vi "MinimalHost_FPGA_TEST.vi"() -> ()   [LabVIEW 2018]
uses:
  <vilib>/rvi/interface/nirviOpenFPGA/nirviOpenFPGA.xnode
  <vilib>/rvi/interface/nirviReadWriteControl/nirviReadWriteControl.xnode
  <vilib>/rvi/interface/Simulation/niFpgaSimulationCallBeginRW.vi
  <vilib>/rvi/errors/niLvFpgaAdjustHostInterfaceError.vi
  ProjectFiles/FPGA Bitfiles/FPGALoopCountTest_3.lvbitx
  TestCode/FPGA_LoopCount_Test.vi
panel:
  out "error out 2":errorcluster
  out "Configuration Error 2":bool
  out "Configured? 2":bool
  out "SPI Idle":bool
  out "LoopCount":i32
  out "error out":errorcluster
  out "IO Module\\Initialization Done":bool
  out "FPGA Probe":i16
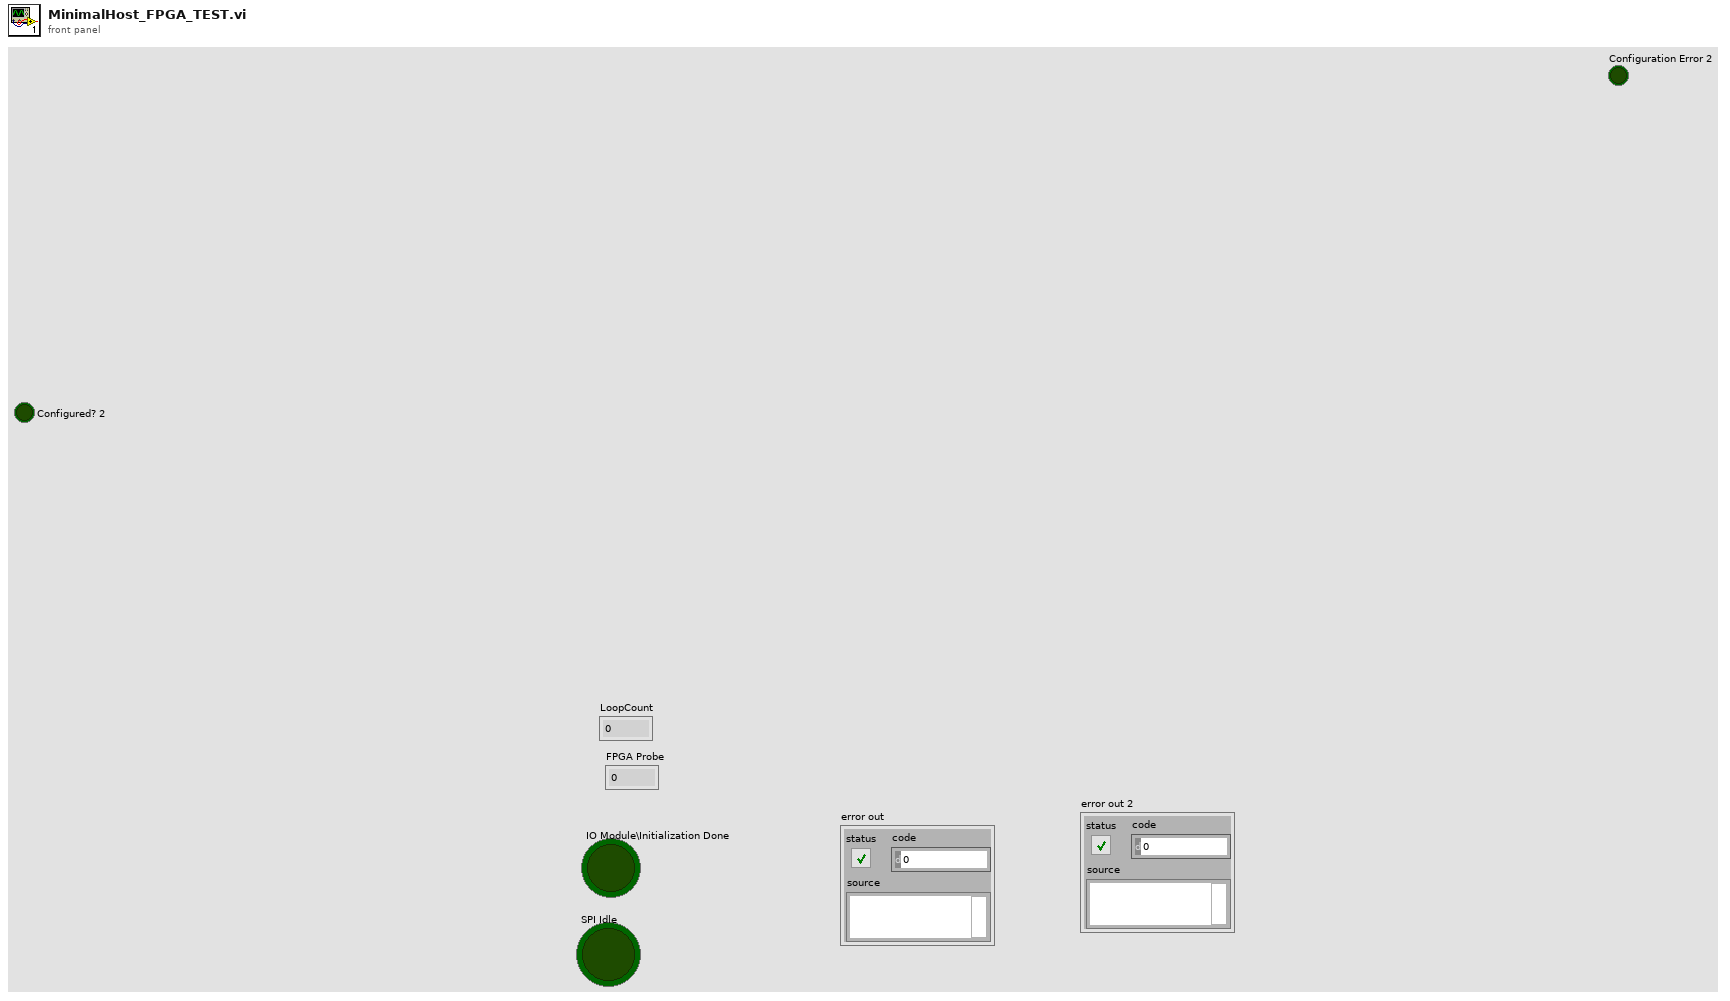
[diagram p1: front panel]
types:
  T1 = enum8{"Internal Clock PLL Off", "Internal Clock PLL On (CLK_IN)", "External Clock (CLK_IN)", "Internal Clock PLL On (IoModSyncClk)"}
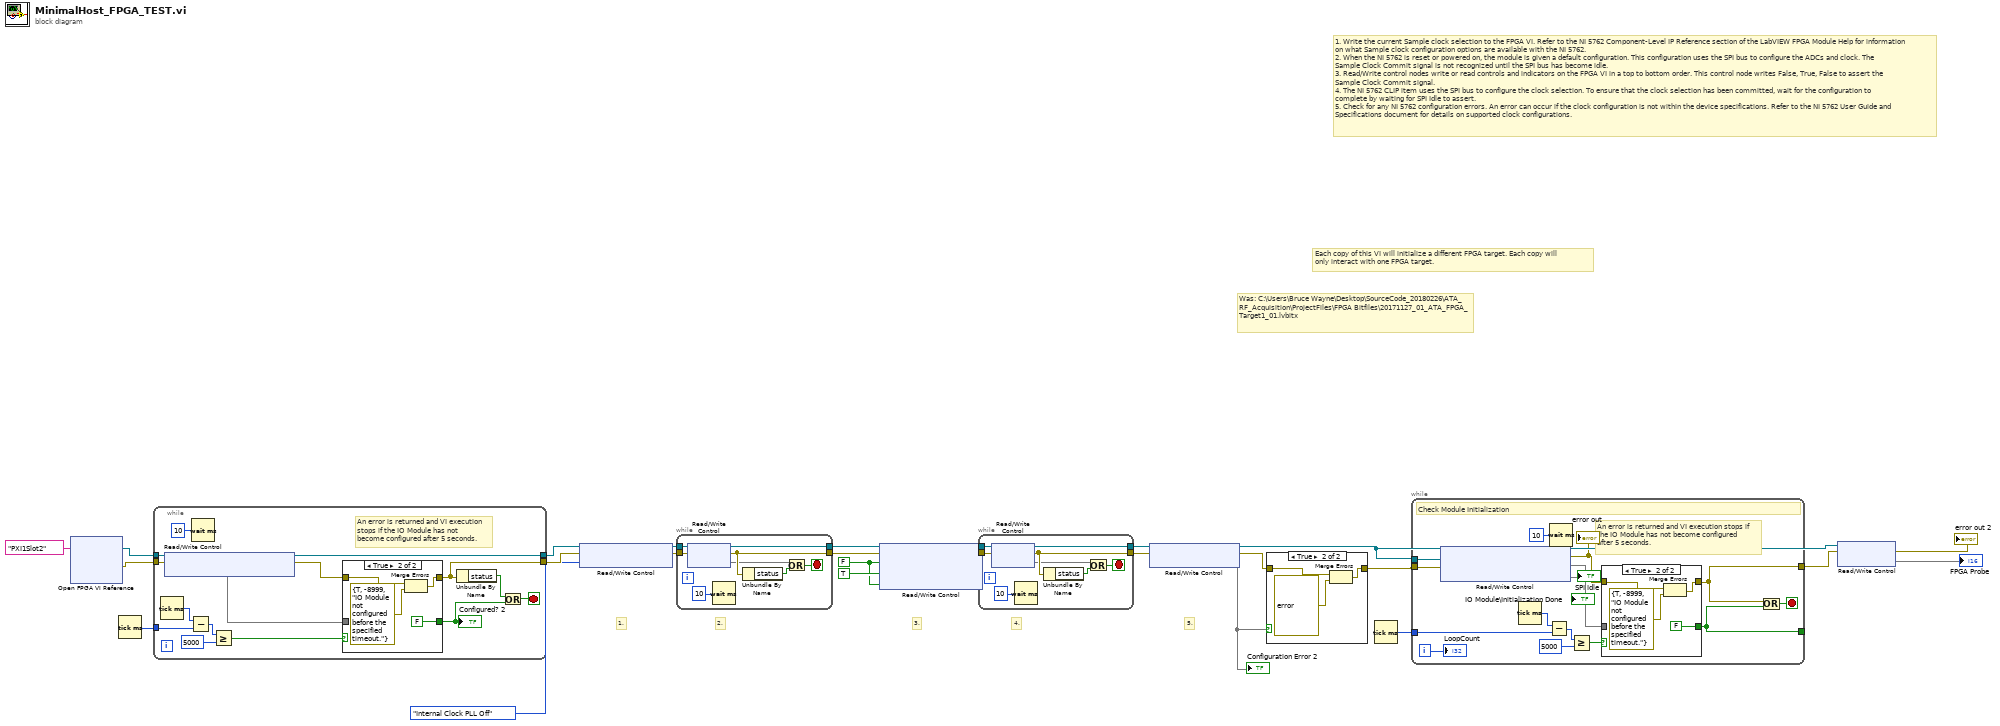
[diagram p0: block diagram]
diagram:
  w15 = FALSE ("Sample Clock Commit")
  # "1. Write the current Sample clock selection to the FPGA VI. Refer to the NI 5762 Component-Level IP Reference section of the LabVIEW FPGA Module Help for information on what Sample clock configuration options are available with the NI 5762.\n2. When the NI 5762 is reset or powered on, the module is given a default configuration. This configuration uses the SPI bus to configure the ADCs and clock. The Sample Clock Commit signal is not recognized until the SPI bus has become idle.\n3. Read/Write control nodes write or read controls and indicators on the FPGA VI in a top to bottom order. This control node writes False, True, False to assert the Sample Clock Commit signal.\n4. The NI 5762 CLIP item uses the SPI bus to configure the clock selection. To ensure that the clock selection has been committed, wait for the configuration to complete by waiting for SPI Idle to assert.\n5. Check for any NI 5762 configuration errors. An error can occur if the clock configuration is not within the device specifications. Refer to the NI 5762 User Guide and Specifications document for details on supported clock configurations."
  # "5."
  # "4."
  # "3."
  # "2."
  # "1."
  # "Was: C:\\Users\\Bruce Wayne\\Desktop\\SourceCode_20180226\\ATA_RF_Acquisition\\ProjectFiles\\FPGA Bitfiles\\20171127_01_ATA_FPGA_Target1_01.lvbitx"
  # "Each copy of this VI will initialize a different FPGA target. Each copy will\nonly interact with one FPGA target."
  n1 = xnode ("Open FPGA VI Reference")("resource name"=tag "PXI1Slot2") -> ("FPGA VI Reference Out"=w8:refnum<k20>, "error out"=w7:errorcluster)  [unwired: 1 in]
  n2 = Tick Count (ms)() -> (millisecond timer value=w21:u32)
  n3 = while {
    tunnel: w7 -> [w33]
    tunnel: [w37] -> w6
    tunnel: [w29] -> w5
    tunnel: w8 -> [w32]
    tunnel: w21 -> [w27]
    stop <- w35 stop-if-true
    # "An error is returned and VI execution stops if the IO Module has not become configured after 5 seconds."
    n4 = Tick Count (ms)() -> (millisecond timer value=w28:u32)
    n5 = xnode "Read/Write Control"("FPGA VI Reference In"=w32, "error in"=w33) -> ("FPGA VI Reference Out"=w29:refnum<k20>, "error out"=w30:errorcluster, "IO Module\\Initialization Done"=w31)
    n6 = Subtract(x=w28, y=w27) -> (x-y=w26:u32)
    n7 = Wait (ms)(milliseconds to wait=u32 10) -> ()  [unwired: 1 out]
    n8 = Greater Or Equal?(x=w26, y=u32 5000) -> (x >= y?=w38:bool)
    n9 = case shown="True" w38 {
      tunnel: [w42 FALSE ("Configured?")] -> w34
      tunnel: w31 -> [w42 _]
      tunnel: [w41 w45] -> w37
      tunnel: w30 -> [w41 w43]
      frame False {
      }
      frame True {
        n10 = Merge Errors(w43, errorcluster {"status"=TRUE, "code"=-8999, "source"="IO Module not configured before the specified timeout."} ("error in")) -> (w45:errorcluster)
      }
    }
    "Configured? 2" <- w34
    n11 = Unbundle By Name(w37) -> ("status"=w36:bool)
    n12 = Or(x=w36, y=w34) -> (x .or. y?=w35:bool)
  }
  n13 = xnode "Read/Write Control"("FPGA VI Reference In"=w5, "error in"=w6, "Sample Clock Select"=T1."Internal Clock PLL Off" ("Clock Source 2")) -> ("FPGA VI Reference Out"=w9:refnum<k20>, "error out"=w10:errorcluster)
  n14 = while {
    tunnel: w9 -> [w50]
    tunnel: w10 -> [w51]
    tunnel: [w48] -> w12
    tunnel: [w49] -> w11
    stop <- w52 stop-if-true
    n15 = xnode "Read/Write Control"("FPGA VI Reference In"=w50, "error in"=w51) -> ("FPGA VI Reference Out"=w49:refnum<k20>, "error out"=w48:errorcluster, "SPI Idle"=w47)
    n16 = Wait (ms)(milliseconds to wait=u32 10) -> ()  [unwired: 1 out]
    n17 = Unbundle By Name(w48) -> ("status"=w53:bool)
    n18 = Or(x=w47, y=w53) -> (x .or. y?=w52:bool)
  }
  n19 = xnode "Read/Write Control"("FPGA VI Reference In"=w11, "error in"=w12, "Sample Clock Commit"=w15, "Sample Clock Commit"=TRUE, "Sample Clock Commit"=w15) -> ("FPGA VI Reference Out"=w13:refnum<k20>, "error out"=w14:errorcluster)
  n20 = while {
    tunnel: w13 -> [w59]
    tunnel: w14 -> [w58]
    tunnel: [w56] -> w18
    tunnel: [w57] -> w17
    stop <- w60 stop-if-true
    n21 = xnode "Read/Write Control"("FPGA VI Reference In"=w59, "error in"=w58) -> ("FPGA VI Reference Out"=w57:refnum<k20>, "error out"=w56:errorcluster, "SPI Idle"=w55)
    n22 = Wait (ms)(milliseconds to wait=u32 10) -> ()  [unwired: 1 out]
    n23 = Unbundle By Name(w56) -> ("status"=w61:bool)
    n24 = Or(x=w55, y=w61) -> (x .or. y?=w60:bool)
  }
  n25 = xnode "Read/Write Control"("FPGA VI Reference In"=w17, "error in"=w18) -> ("FPGA VI Reference Out"=w4:refnum<k20>, "error out"=w19:errorcluster, "Configuration Error"=w20)
  "Configuration Error 2" <- w20
  n26 = case shown="True" w20 {
    tunnel: [w63 w66] -> w3
    tunnel: w19 -> [w63 w64]
    frame False {
    }
    frame True {
      n27 = Merge Errors(w64, errorcluster {"status"=TRUE, "code"=-8998, "source"="IO Module clock not configured correctly. Please ensure that the desired clock meets the required specifications."} ("error in")) -> (w66:errorcluster)
    }
  }
  n28 = Tick Count (ms)() -> (millisecond timer value=w23:u32)
  n29 = while {
    tunnel: [w69] -> w22
    tunnel: w4 -> [w73]
    tunnel: w3 -> [w72]
    tunnel: w23 -> [w71]
    tunnel: [w70] -> _
    i -> [w68]
    stop <- w78 stop-if-true
    # "An error is returned and VI execution stops if the IO Module has not become configured after 5 seconds."
    # "Check Module Initialization"
    n30 = xnode "Read/Write Control"("FPGA VI Reference In"=w73, "error in"=w72) -> ("error out"=w76:errorcluster, "IO Module\\Initialization Done"=w77, "SPI Idle"=→"SPI Idle")  [unwired: 1 out]
    "IO Module\\Initialization Done" <- w77
    "error out" <- w76
    n31 = Tick Count (ms)() -> (millisecond timer value=w75:u32)
    n32 = Subtract(x=w75, y=w71) -> (x-y=w74:u32)
    n33 = Wait (ms)(milliseconds to wait=u32 10) -> ()  [unwired: 1 out]
    n34 = Greater Or Equal?(x=w74, y=u32 5000) -> (x >= y?=w79:bool)
    n35 = case shown="True" w79 {
      tunnel: [w82 FALSE ("Configured?")] -> w70
      tunnel: w77 -> [w82 _]
      tunnel: [w83 w86] -> w69
      tunnel: w76 -> [w83 w84]
      frame False {
      }
      frame True {
        n36 = Merge Errors(w84, errorcluster {"status"=TRUE, "code"=-8999, "source"="IO Module not configured before the specified timeout."} ("error in")) -> (w86:errorcluster)
      }
    }
    n37 = Or(x=w69, y=w70) -> (x .or. y?=w78:bool)
    "LoopCount" <- w68
  }
  n38 = xnode "Read/Write Control"("FPGA VI Reference In"=w4, "error in"=w22) -> ("error out"=→"error out 2":errorcluster, "LoopCount"=→"FPGA Probe")  [unwired: 1 out]
